vi "SetMatlabTemp.vi"(8 "IgnoreContainerName":bool, 10 "Variant":variant, 11 "ExpID":string) -> (0 "Matlab Param Data":T1[](array[typedef]), 3 "index out":dbl)   [LabVIEW 2017]
uses:
  Types/MatlabDataBundle.ctl
  Types/MatlabDataType.ctl
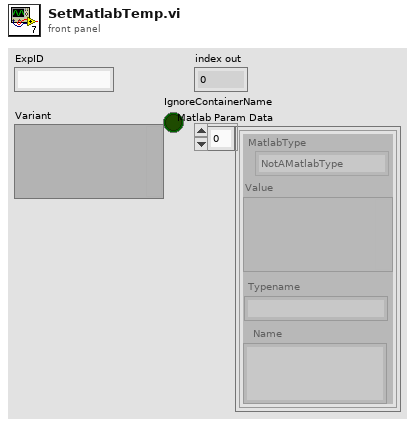
[diagram p1: front panel]
types:
  T1 = typedef "MatlabDataBundle.ctl" = cluster{"MatlabType":T2, "Value":variant, "Name":string, "Typename":string}
  T2 = typedef "MatlabDataType.ctl" = enum16{"NotAMatlabType", "Real", "Complex", "String", "Boolean"}
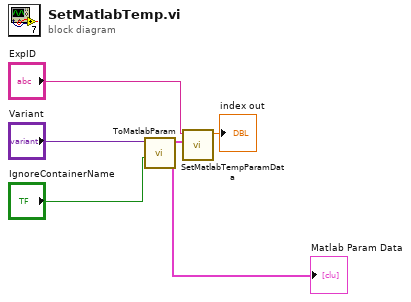
[diagram p0: block diagram]
diagram:
  n1 = call "ToMatlabParam.vi"("IgnoreContainerName"="IgnoreContainerName", "Value"="Variant") -> ("Matlab Param Data"=w2:T1[])  [unwired: 9 in]
  "Matlab Param Data" <- w2
  n2 = call "SetMatlabTempParamData.vi"("Matlab param data"=w2, "ExperimentID"="ExpID") -> ("index out"=→"index out":dbl)  [unwired: 9 in]
